vi "restore_config.vi"   [LabVIEW 2011]
doc: "Restores the chirp pulse experiment settings from a config file."
uses:
  <vilib>/Utility/config.llb/Read Key (I32).vi
  global.vi
  <vilib>/Utility/config.llb/Read Key (Boolean).vi
  <vilib>/Utility/config.llb/Read Key (Double).vi
  <vilib>/Utility/config.llb/Read Key (String).vi
  <vilib>/Utility/config.llb/NI_LVConfig.lvlib
types:
  T1 = typedef "NI_LVConfig.lvlib/Config Data RefNum.ctl" = refnum<k1>
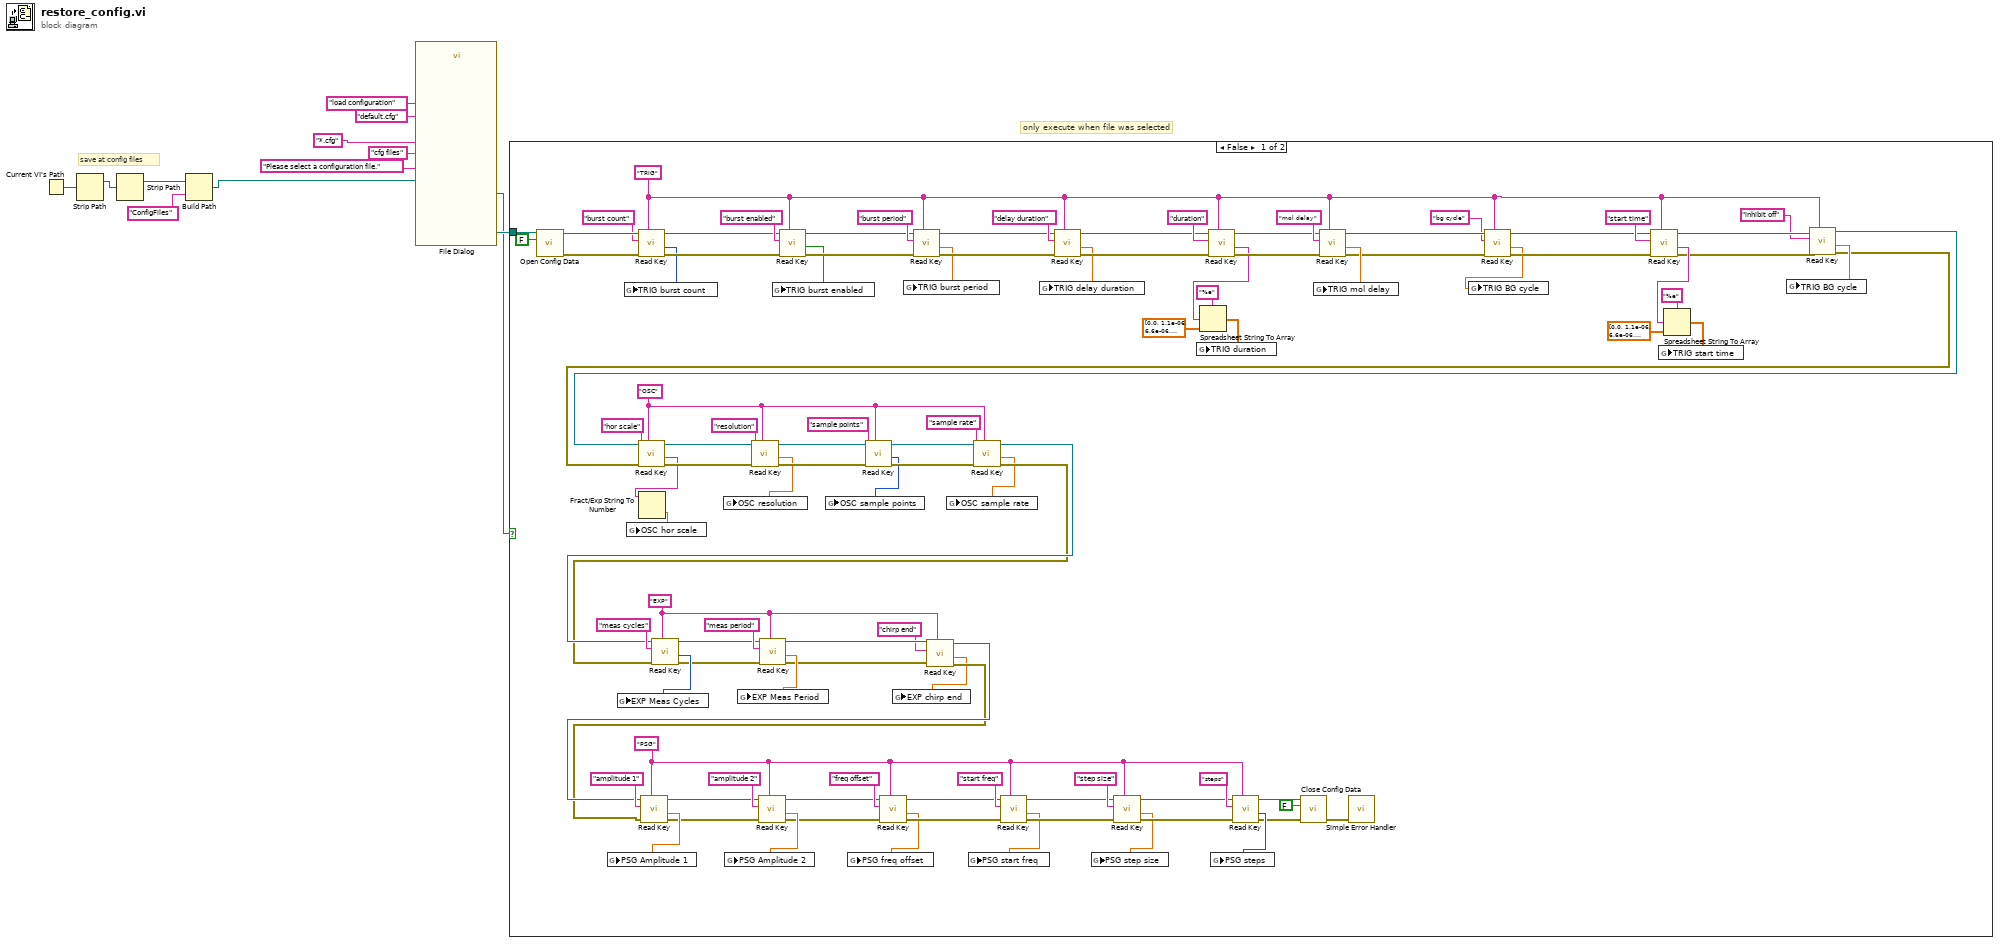
[diagram p0: block diagram]
diagram:
  # "only execute when file was selected"
  # "save at config files"
  n1 = Current VI's Path() -> (path=w6:path)
  n2 = Strip Path(path=w6) -> (stripped path=w4:path)  [unwired: 1 out]
  n3 = Strip Path(path=w4) -> (stripped path=w3:path)  [unwired: 1 out]
  n4 = Build Path(base path=w3, name or relative path="ConfigFiles") -> (appended path=w2:path)
  n5 = call "File Dialog"("start path"=w2, "prompt"="Please select a configuration file.", "button label"="load configuration", "default name"="default.cfg", "pattern (all files)"="*.cfg" ("default name"), "pattern label"="cfg files") -> ("selected path"=w12:path, "cancelled"=w1:bool)  [unwired: 6 in, 2 out]
  n6 = case shown="False" w1 {
    tunnel: w12 -> [w113 _]
    frame False {
      w45 = "PSG"
      w22 = "EXP"
      w86 = "OSC"
      w13 = "TRIG"
      n7 = call <vilib>:"Open Config Data.vi"("create file if necessary (T)"=FALSE, "configuration file path"=w113) -> ("error out"=w116:errorcluster, "refnum"=w117:T1)  [unwired: 1 in, 7 out]
      n8 = call-poly <vilib>:"Read Key.vi"("section"=w13, "error in (no error)"=w116, "key"="burst count" ("Key 1"), "refnum"=w117) -> ("error out"=w104:errorcluster, "value"=w71:i32, "refnum out"=w108:T1)  [unwired: 4 in, 1 out]
      n9 = global write "global.vi" "TRIG burst count"(w71) -> ()
      n10 = call-poly <vilib>:"Read Key.vi"("section"=w13, "error in (no error)"=w104, "key"="burst enabled" ("Key 1"), "refnum"=w108) -> ("error out"=w103:errorcluster, "value"=w70:bool, "refnum out"=w107:T1)  [unwired: 4 in, 1 out]
      n11 = global write "global.vi" "TRIG burst enabled"(w70) -> ()
      n12 = call-poly <vilib>:"Read Key.vi"("section"=w13, "error in (no error)"=w103, "key"="burst period" ("Key 1"), "refnum"=w107) -> ("error out"=w102:errorcluster, "value"=w69:dbl, "refnum out"=w106:T1)  [unwired: 4 in, 1 out]
      n13 = global write "global.vi" "TRIG burst period"(w69) -> ()
      n14 = call-poly <vilib>:"Read Key.vi"("section"=w13, "error in (no error)"=w102, "key"="delay duration" ("Key 1"), "refnum"=w106) -> ("error out"=w101:errorcluster, "value"=w68:dbl, "refnum out"=w105:T1)  [unwired: 4 in, 1 out]
      n15 = global write "global.vi" "TRIG delay duration"(w68) -> ()
      n16 = call-poly <vilib>:"Read Key.vi"("section"=w13, "error in (no error)"=w101, "key"="duration" ("Key 1"), "refnum"=w105) -> ("error out"=w97:errorcluster, "value"=w65:string, "refnum out"=w98:T1)  [unwired: 4 in, 1 out]
      n17 = Spreadsheet String To Array(format string="%e", spreadsheet string=w65, array type (2D Dbl)=dbl[] [0.0, 1.1e-06, 6.6e-06, 6.4e-06] ("TRIG start time")) -> (array=w66:dbl[])  [unwired: 1 in]
      n18 = global write "global.vi" "TRIG duration"(w66) -> ()
      n19 = call-poly <vilib>:"Read Key.vi"("section"=w13, "error in (no error)"=w97, "key"="mol delay" ("Key 1"), "refnum"=w98) -> ("error out"=w30:errorcluster, "value"=w60:dbl, "refnum out"=w29:T1)  [unwired: 4 in, 1 out]
      n20 = global write "global.vi" "TRIG mol delay"(w60) -> ()
      n21 = call-poly <vilib>:"Read Key.vi"("section"=w13, "error in (no error)"=w30, "key"="bg cycle" ("Key 1"), "refnum"=w29) -> ("error out"=w31:errorcluster, "value"=w27:dbl, "refnum out"=w32:T1)  [unwired: 4 in, 1 out]
      n22 = global write "global.vi" "TRIG BG cycle"(w27) -> ()
      n23 = call-poly <vilib>:"Read Key.vi"("section"=w13, "error in (no error)"=w31, "key"="start time" ("Key 1"), "refnum"=w32) -> ("error out"=w18:errorcluster, "value"=w59:string, "refnum out"=w19:T1)  [unwired: 4 in, 1 out]
      n24 = Spreadsheet String To Array(format string="%e", spreadsheet string=w59, array type (2D Dbl)=dbl[] [0.0, 1.1e-06, 6.6e-06, 6.4e-06] ("TRIG start time")) -> (array=w62:dbl[])  [unwired: 1 in]
      n25 = global write "global.vi" "TRIG start time"(w62) -> ()
      n26 = call-poly <vilib>:"Read Key.vi"("section"=w13, "error in (no error)"=w18, "key"="inhibit off" ("Key 1"), "refnum"=w19) -> ("error out"=w14:errorcluster, "value"=w16:dbl, "refnum out"=w15:T1)  [unwired: 4 in, 1 out]
      n27 = call-poly <vilib>:"Read Key.vi"("section"=w86, "error in (no error)"=w14, "key"="hor scale" ("Key 1"), "refnum"=w15) -> ("error out"=w91:errorcluster, "value"=w38:string, "refnum out"=w93:T1)  [unwired: 4 in, 1 out]
      n28 = Fract/Exp String To Number(string=w38) -> (number=w37:dbl)  [unwired: 3 in, 1 out]
      n29 = global write "global.vi" "OSC hor scale"(w37) -> ()
      n30 = call-poly <vilib>:"Read Key.vi"("section"=w86, "error in (no error)"=w91, "key"="resolution" ("Key 1"), "refnum"=w93) -> ("error out"=w90:errorcluster, "value"=w58:dbl, "refnum out"=w92:T1)  [unwired: 4 in, 1 out]
      n31 = global write "global.vi" "OSC resolution"(w58) -> ()
      n32 = call-poly <vilib>:"Read Key.vi"("section"=w86, "error in (no error)"=w90, "key"="sample points" ("Key 1"), "refnum"=w92) -> ("error out"=w87:errorcluster, "value"=w57:i32, "refnum out"=w88:T1)  [unwired: 4 in, 1 out]
      n33 = global write "global.vi" "OSC sample points"(w57) -> ()
      n34 = call-poly <vilib>:"Read Key.vi"("section"=w86, "error in (no error)"=w87, "key"="sample rate" ("Key 1"), "refnum"=w88) -> ("error out"=w83:errorcluster, "value"=w56:dbl, "refnum out"=w84:T1)  [unwired: 4 in, 1 out]
      n35 = call-poly <vilib>:"Read Key.vi"("section"=w22, "error in (no error)"=w83, "key"="meas cycles" ("Key 1"), "refnum"=w84) -> ("error out"=w34:errorcluster, "value"=w55:i32, "refnum out"=w35:T1)  [unwired: 4 in, 1 out]
      n36 = global write "global.vi" "EXP Meas Cycles"(w55) -> ()
      n37 = call-poly <vilib>:"Read Key.vi"("section"=w22, "error in (no error)"=w34, "key"="meas period" ("Key 1"), "refnum"=w35) -> ("error out"=w24:errorcluster, "value"=w33:dbl, "refnum out"=w23:T1)  [unwired: 4 in, 1 out]
      n38 = global write "global.vi" "EXP Meas Period"(w33) -> ()
      n39 = call-poly <vilib>:"Read Key.vi"("section"=w22, "error in (no error)"=w24, "key"="chirp end", "refnum"=w23) -> ("error out"=w25:errorcluster, "value"=w21:dbl, "refnum out"=w26:T1)  [unwired: 4 in, 1 out]
      n40 = call-poly <vilib>:"Read Key.vi"("section"=w45, "error in (no error)"=w25, "key"="amplitude 1" ("Key 1"), "refnum"=w26) -> ("error out"=w40:errorcluster, "value"=w48:dbl, "refnum out"=w42:T1)  [unwired: 4 in, 1 out]
      n41 = global write "global.vi" "PSG Amplitude 1"(w48) -> ()
      n42 = call-poly <vilib>:"Read Key.vi"("section"=w45, "error in (no error)"=w40, "key"="amplitude 2" ("Key 1"), "refnum"=w42) -> ("error out"=w39:errorcluster, "value"=w46:dbl, "refnum out"=w41:T1)  [unwired: 4 in, 1 out]
      n43 = global write "global.vi" "PSG Amplitude 2"(w46) -> ()
      n44 = call-poly <vilib>:"Read Key.vi"("section"=w45, "error in (no error)"=w39, "key"="freq offset" ("Key 1"), "refnum"=w41) -> ("error out"=w77:errorcluster, "value"=w54:dbl, "refnum out"=w79:T1)  [unwired: 4 in, 1 out]
      n45 = global write "global.vi" "PSG freq offset"(w54) -> ()
      n46 = global write "global.vi" "EXP chirp end"(w21) -> ()
      n47 = global write "global.vi" "OSC sample rate"(w56) -> ()
      n48 = call-poly <vilib>:"Read Key.vi"("section"=w45, "error in (no error)"=w77, "key"="start freq" ("Key 1"), "refnum"=w79) -> ("error out"=w76:errorcluster, "value"=w53:dbl, "refnum out"=w78:T1)  [unwired: 4 in, 1 out]
      n49 = global write "global.vi" "PSG start freq"(w53) -> ()
      n50 = call-poly <vilib>:"Read Key.vi"("section"=w45, "error in (no error)"=w76, "key"="step size" ("Key 1"), "refnum"=w78) -> ("error out"=w73:errorcluster, "value"=w52:dbl, "refnum out"=w74:T1)  [unwired: 4 in, 1 out]
      n51 = global write "global.vi" "PSG step size"(w52) -> ()
      n52 = call-poly <vilib>:"Read Key.vi"("section"=w45, "error in (no error)"=w73, "key"="steps" ("Key 1"), "refnum"=w74) -> ("error out"=w43:errorcluster, "value"=w51:i32, "refnum out"=w44:T1)  [unwired: 4 in, 1 out]
      n53 = global write "global.vi" "PSG steps"(w51) -> ()
      n54 = call <vilib>:"Close Config Data.vi"("error in (no error)"=w43, "write file if changed (T)"=FALSE, "refnum"=w44) -> ("error out"=w114:errorcluster)  [unwired: 8 out]
      n55 = call <vilib>:"Simple Error Handler.vi"("error in (no error)"=w114) -> ()  [unwired: 1 in, 8 out]
      n56 = global write "global.vi" "TRIG BG cycle"(w16) -> ()
    }
    frame True {
    }
  }
